vi "Read Measurement.vi"(8 "error in (no error)":errorcluster, 9 "Actual Unit (F: Base unit)":bool, 10 "Immediately  (F: Wait for stable result)":bool, 11 "VISA resource name":refnum<visa-resource-name>) -> (0 "error out":errorcluster, 1 "Unit":string, 2 "Value":dbl, 3 "VISA resource name out":refnum<visa-resource-name>, 4 "Stability Sign":string="-")   [LabVIEW 2017, in "RadWag balances and scales.lvlib"]
doc: "Returns current value of weight.\nDepending on configuration it can wait for stable reasult or return result immediatly.\nResult can be returned in balance base unit (g) or in acctual unit (oz., mg, no. of pieces, etc.)"
uses:
  <instrlib>/Prev/RadWag Continuous Read Folder/RadWag balances and scales.lvlib
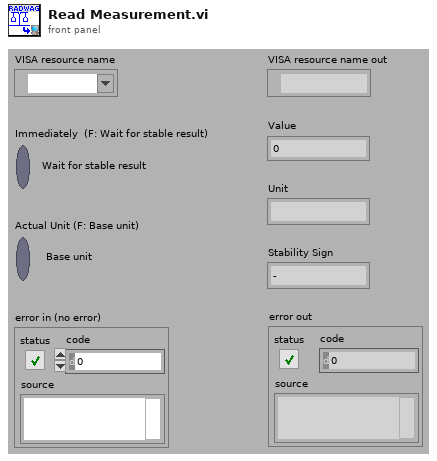
[diagram p1: front panel]
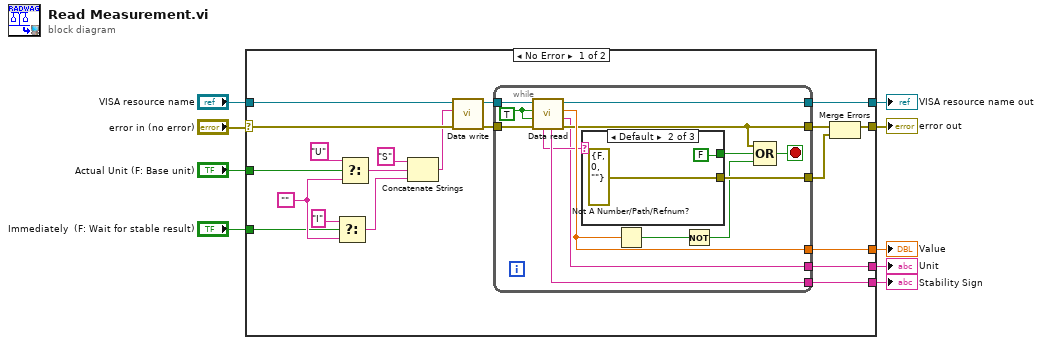
[diagram p0: block diagram]
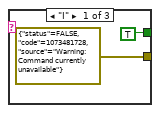
[diagram p2: hidden frame]
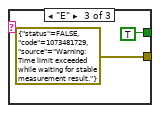
[diagram p3: hidden frame]
diagram:
  n1 = case shown="No Error" "error in (no error)" {
    selector: "error in (no error)" -> [w22 w50]
    tunnel: "VISA resource name" -> [w29 w51]
    tunnel: "Immediately  (F: Wait for stable result)" -> [w13 _]
    tunnel: "Actual Unit (F: Base unit)" -> [w14 _]
    tunnel: [w26 w51] -> w5
    tunnel: [w11 w50] -> w4
    tunnel: [w25 _] -> w3
    tunnel: [w24 _] -> w2
    tunnel: [w23 _] -> w1
    frame No Error {
      w19 = ""
      n2 = Select(t="I", s=w13, f=w19) -> (s? t:f=w17:string)
      n3 = Select(t="U", s=w14, f=w19) -> (s? t:f=w18:string)
      n4 = Concatenate Strings("S" ("ID"), w18, w17) -> (w20:string)
      n5 = call <instrlib>:"Data write.vi"("error in (no error)"=w22, "ID"=w20, "VISA resource name"=w29) -> ("error out"=w27:errorcluster, "VISA resource name out"=w28:refnum<visa-resource-name>)  [unwired: 7 in]
      n6 = while {
        tunnel: w28 -> [w43]
        tunnel: w27 -> [w42]
        tunnel: [w41] -> w26
        tunnel: [w35] -> w12
        tunnel: [w38] -> w25
        tunnel: [w31] -> w24
        tunnel: [w37] -> w23
        tunnel: [w33] -> w10
        stop <- w40 stop-if-true
        w36 = TRUE ("Stability sign?")
        n7 = call <instrlib>:"Data read.vi"("error in (no error)"=w42, "Data With Stability Sign"=w36, "Decode Status (F)/ Decode Data (T)"=w36, "VISA resource name"=w43) -> ("error out"=w35:errorcluster, "Unit"=w31:string, "Value"=w38:dbl, "VISA resource name out"=w41:refnum<visa-resource-name>, "Stability Sign"=w37:string, "Status"=w34:string)  [unwired: 1 in, 1 out]
        n8 = case shown="Default" w34 {
          tunnel: [errorcluster {"status"=FALSE, "code"=1073481728, "source"="Warning: Command currently unavailable"} ("t") errorcluster {"status"=FALSE, "code"=0, "source"=""} ("error constant") errorcluster {"status"=FALSE, "code"=1073481729, "source"="Warning: Time limit exceeded while waiting for stable measurement result."} ("t")] -> w33
          tunnel: [TRUE FALSE TRUE] -> w32
          frame "I" {
          }
          frame Default {
          }
          frame "E" {
          }
        }
        n9 = Not A Number/Path/Refnum?(number/path/refnum=w38) -> (NaN/Path/Refnum?=w39:bool)
        n10 = Not(x=w39) -> (.not. x?=w30:bool)
        n11 = Compound Arithmetic op=OR(w35, w32, w30) -> (w40:bool)
      }
      n12 = Merge Errors(w12, w10) -> (w11:errorcluster)
    }
    frame Error {
    }
  }
  "VISA resource name out" <- w5
  "error out" <- w4
  "Stability Sign" <- w1
  "Value" <- w3
  "Unit" <- w2
